vi "Crear Conexion.vi"(8 "error in (no error)":errorcluster, 11 "CYPRESS in":refnum<class "CYPRESS.lvclass">) -> (0 "error out":errorcluster, 3 "CYPRESS out":refnum<class "CYPRESS.lvclass">)   [LabVIEW 2019, in "CYPRESS.lvclass"]
uses:
  CYPRESS.lvclass
  CYPRESS.lvclass/CYPRESS.ctl
  <vilib>/Instr/_visa.llb/VISA Configure Serial Port (Instr).vi
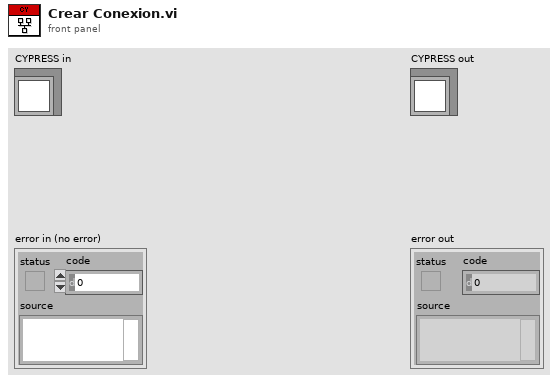
[diagram p1: front panel]
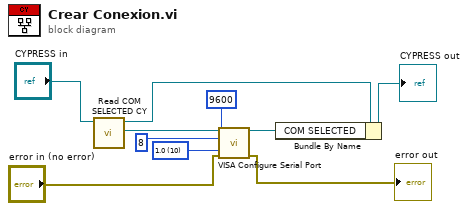
[diagram p0: block diagram]
diagram:
  w4 = u16 10 items=["1.0"=10, "1.5"=15, "2.0"=20] ("stop bits (10: 1 bit)")
  n1 = call "Read COM SELECTED CY.vi"("TI in"="CYPRESS in") -> ("COM SELECTED"=w3:refnum<visa-resource-name>, "TI out"=w1:refnum<class "CYPRESS.lvclass">)  [unwired: 8 in, 1 out]
  n2 = call-poly "VISA Configure Serial Port"("VISA resource name"=w3, "baud rate (9600)"=u32 9600, "data bits (8)"=u16 8, "error in (no error)"="error in (no error)", "stop bits (10: 1 bit)"=w4) -> ("VISA resource name out"=w5:refnum<visa-resource-name>, "error out"=→"error out":errorcluster)  [unwired: 9 in]
  n3 = Bundle By Name(cluster=w1, "COM SELECTED"=w5) -> (→"CYPRESS out":refnum<class "CYPRESS.lvclass">)
